vi "StoeDisplayImagesReference.vi"(0 "object in":refnum<class "Hamamatsu.lvclass">, 2 "Image Src":T1[](array[typedef]), 5 "error in (no error)":errorcluster) -> (14 "object out":refnum<class "Hamamatsu.lvclass">, 16 "Images for Display Purpose":T1[](array[typedef]), 19 "error out":errorcluster)   [LabVIEW 2021, in "Hamamatsu.lvclass"]
uses:
  Hamamatsu.lvclass
  <vilib>/vision/Image Controls.llb/IMAQ Image.ctl
  Hamamatsu.lvclass/Hamamatsu.ctl
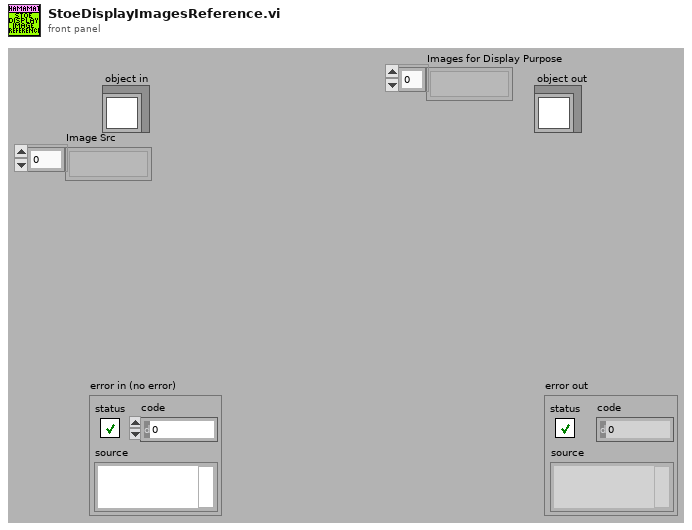
[diagram p1: front panel]
types:
  T1 = typedef "IMAQ Image.ctl" = refnum<image>
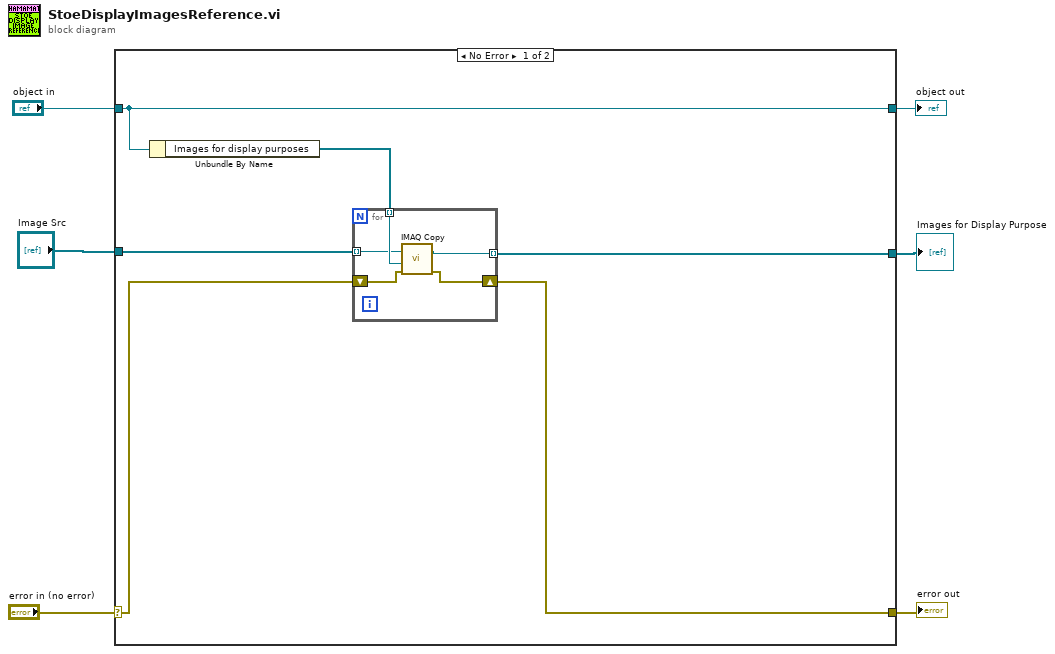
[diagram p0: block diagram]
diagram:
  n1 = case shown="No Error" "error in (no error)" {
    selector: "error in (no error)" -> [w9 w19]
    tunnel: [w8 w19] -> w5
    tunnel: [w12 w18] -> w3
    tunnel: "object in" -> [w12 w18]
    tunnel: "Image Src" -> [w10 _]
    tunnel: [w7 _] -> w1
    frame No Error {
      n2 = Unbundle By Name(w12) -> ("Images for display purposes"=w11:T1[])
      n3 = for {
        tunnel: w11 -> [w17] mode=indexing
        tunnel: w10 -> [w16] mode=indexing
        shift-right: [w14] -> w8
        shift-left: w9 -> [w15]
        tunnel: [w13] -> w7 mode=indexing
        n4 = call "IMAQ Copy"("error in (no error)"=w15, "Image Dst"=w17, "Image Src"=w16) -> ("error out"=w14:errorcluster, "Image Dst Out"=w13:T1)  [unwired: 3 in]
      }
    }
    frame Error {
    }
  }
  "error out" <- w5
  "object out" <- w3
  "Images for Display Purpose" <- w1
